vi "Define Mask.vi"(8 "error in (no error)":errorcluster, 11 "FPGA Image":T3(plugin-control)=refnum) -> (0 "error out":errorcluster)   [LabVIEW 2013]
doc: "GUI for selecting a part type and starting a batch process\nPart types list is passed in from caller.\nReturns when Start or Cancel is pressed."
uses:
  Sectors/Number of Wing Sector.ctl
  Mask ROI FG Enum.ctl
  Mask ROI Cluster.ctl
  Common/File IO/INI/Read write mode.ctl
  Message Passing/MsgQ Loops enum.ctl
  System Status/Status FG Enum.ctl
  Common/State Machines/State Machine Lib.lvlib
  Common/GUI/GUI.lvlib
  <vilib>/vision/NI_Vision_Development_Module.lvlib
  Image Processing.lvlib
  Message Passing/Main MsgQ.lvlib
panel:
  in  "Calculate BG":bool
  in  "Load Current Mask":bool
  out "Right ROI":T1 {"Contours"."Type" items=["No Selection", "Point", "Line", "Rectangle", "Oval", "Polygon", "Freehand Region", "Annulus", "Unused2", "Unused3", "Broken Line", "Freehand Line", "Rotated Rectangle"]}
  out "Left ROI":T1 {"Contours"."Type" items=["No Selection", "Point", "Line", "Rectangle", "Oval", "Polygon", "Freehand Region", "Annulus", "Unused2", "Unused3", "Broken Line", "Freehand Line", "Rotated Rectangle"]}
  out "[Avg BG]":dbl[](array[numeric])
  in  "NumWingSectors":T2=1 items=["1"=1, "2"=2, "4"=4, "8"=8, "16"=16]
  out "State":string
  in  "Exit":bool
  in  "Save Mask":bool
  out "combo mask":T3(plugin-control)
  out "right mask":T3(plugin-control)
  out "right masked image":T3(plugin-control)
  out "right annulus":T4={"Center X"=929, "Center Y"=663, "Inner Radius"=200, "Outer Radius"=405, "Start Angle"=90.0, "End Angle"=180.0} {"End Angle" format="%.2f"; "Start Angle" format="%.2f"; "Center X" scale=0.0..1024.0}
  out "left mask":T3(plugin-control)
  out "left masked image":T3(plugin-control)
  out "left annulus":T4={"Center X"=929, "Center Y"=663, "Inner Radius"=200, "Outer Radius"=405, "Start Angle"=90.0, "End Angle"=180.0} {"End Angle" format="%.2f"; "Start Angle" format="%.2f"; "Center X" scale=0.0..1024.0}
  in  "Accept Threshold":bool
  out "Processed Image":T3(plugin-control)
  in  "Threshold Range":cluster{"Lower value":dbl, "Upper value":dbl}={"Lower value"=106.82432432432432, "Upper value"=255.0} {"Upper value" min=0.0 max=255.0 scale=0.0..255.0; "Lower value" min=0.0 max=255.0 scale=0.0..255.0}
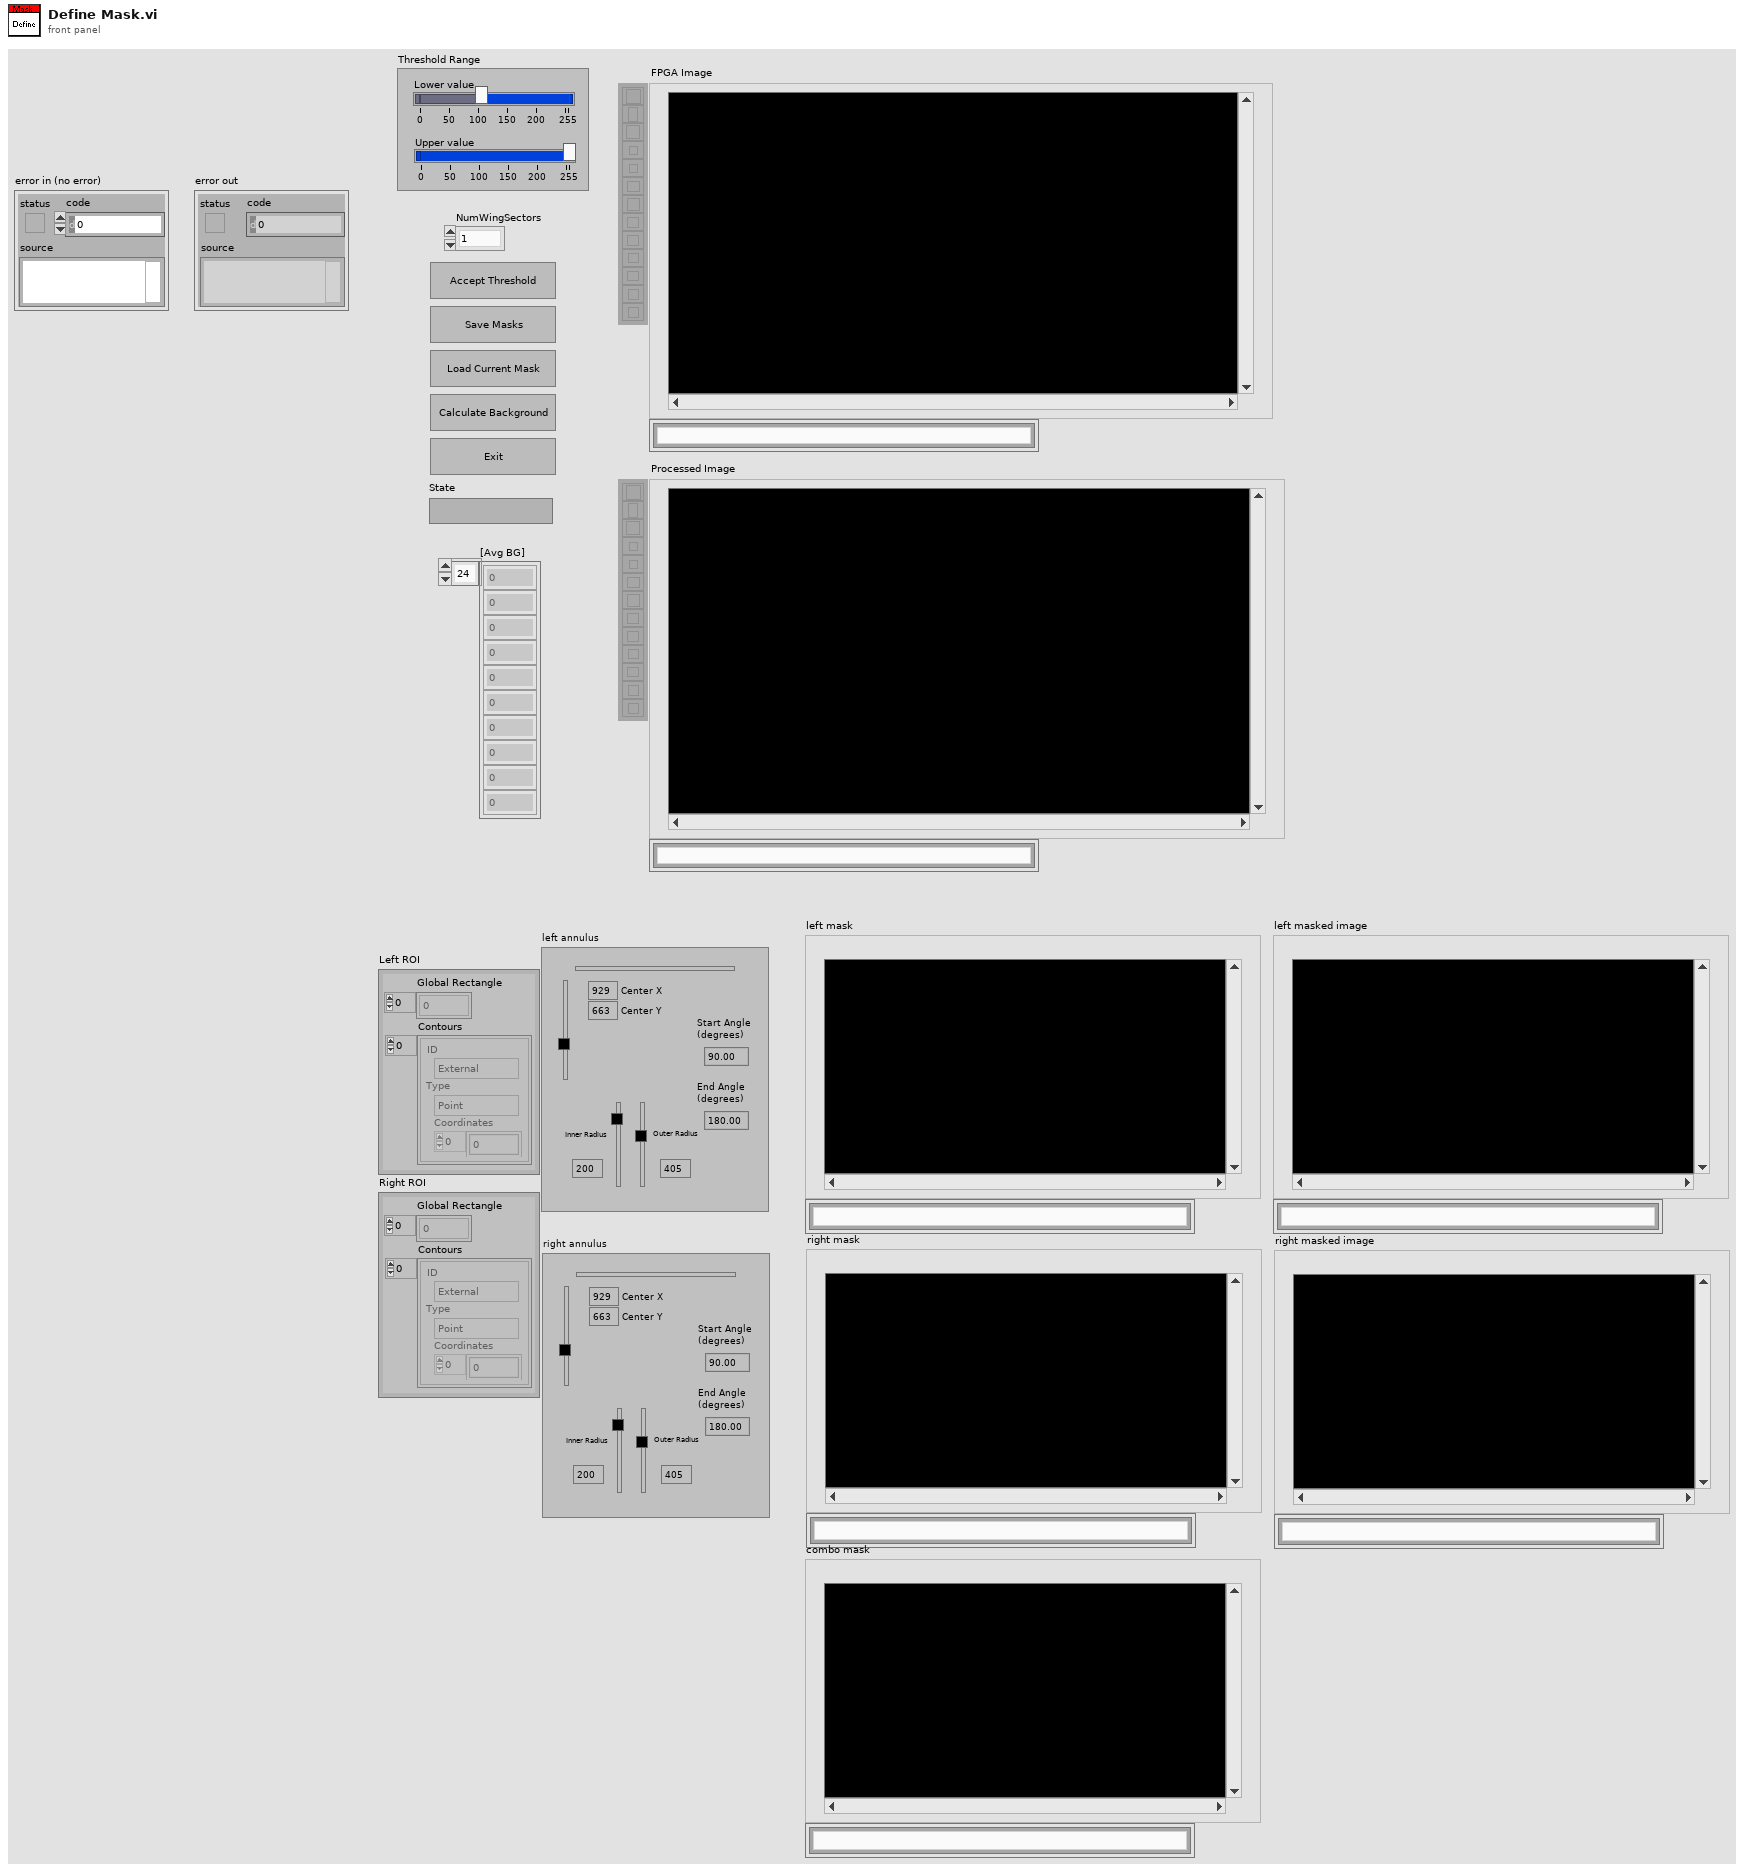
[diagram p1: front panel]
types:
  T1 = typedef "ROI Descriptor" = cluster{"Global Rectangle":i32[], "Contours":cluster{"ID":enum32{"External", "Internal"}, "Type":u32, "Coordinates":i32[]}[]}
  T2 = typedef "Number of Wing Sector.ctl" = u8
  T3 = typedef "IMAQ Image.ctl" = refnum<image>
  T4 = typedef "IMAQ Circle" = cluster{"Center X":i32, "Center Y":i32, "Inner Radius":i32, "Outer Radius":i32, "Start Angle":dbl, "End Angle":dbl}
  T5 = typedef "State Machine Lib.lvlib/STATE cluster.ctl" = cluster{"State":string, "Parameters":variant}
  T6 = typedef "Mask ROI FG Enum.ctl" = enum16{"Read", "Write"}
  T7 = typedef "Main MsgQ.lvlib/MsgQ Loops enum.ctl" = enum16{"User Interface", "Image Acq"}
  T8 = typedef "Read write mode.ctl" = enum16{"Read", "Write"}
  T9 = typedef "Mask ROI Cluster.ctl" = cluster{"left annulus":T4, "right annulus":T4, "Threshold Range":cluster{"Lower value":dbl, "Upper value":dbl}, "[Avg BG]":u8[], "Number of Sectors":u8, "Left ROI":T1, "Right ROI":T1, "Left Start Angle Duty Cycle":fxp<+,8,0>, "Left End Angle Duty Cycle":fxp<+,8,0>, "Right End Angle Duty Cycle":fxp<+,8,0>, "Right Start Angle Duty Cycle":fxp<+,8,0>, "[Sector ROIs]":T1[]}
  T10 = typedef "Status FG Enum.ctl" = enum16{"Reset", "Read", "Write"}
  T11 = typedef "Sector Parameter Cluster.ctl" = cluster{"Start Angle":fxp<+/-,17,2>, "End Angle":fxp<+/-,17,2>, "Inner Radius":u16, "Outter Radius":u16, "Hinge X":u16, "Hinge Y":u16, "NumWingSectors":u8}
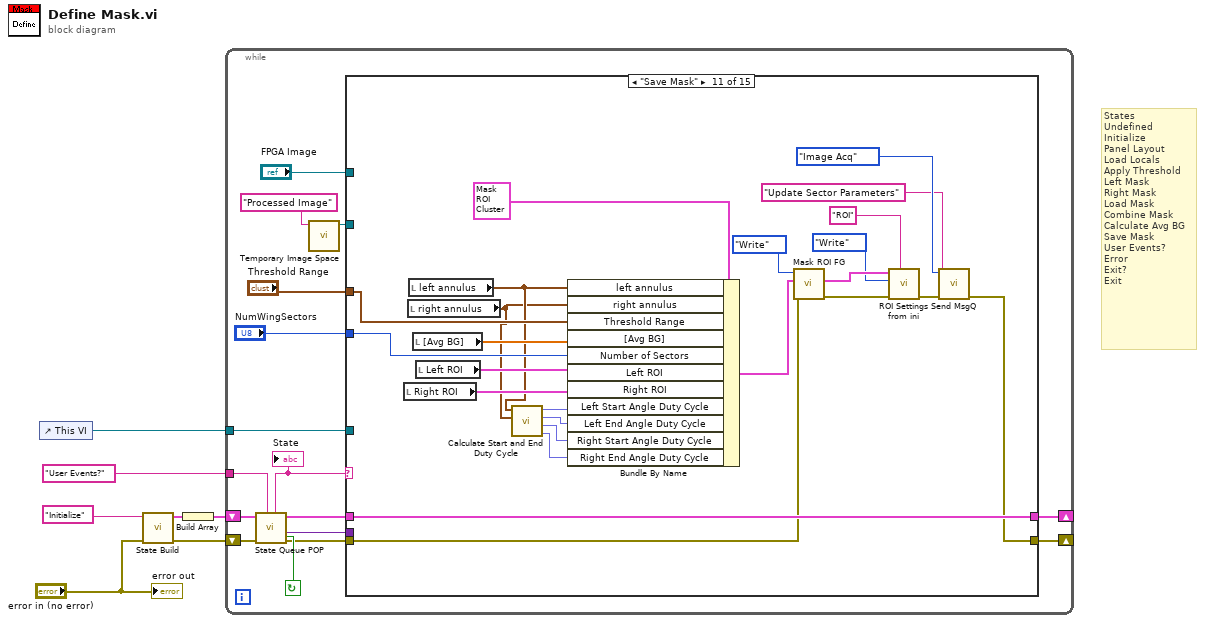
[diagram p0: block diagram]
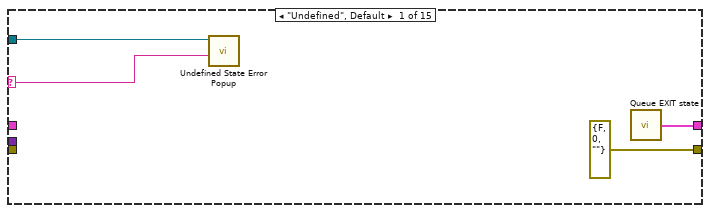
[diagram p2: hidden frame]
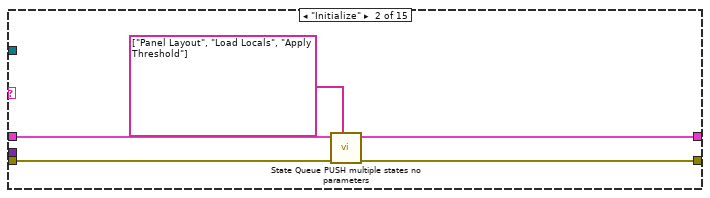
[diagram p3: hidden frame]
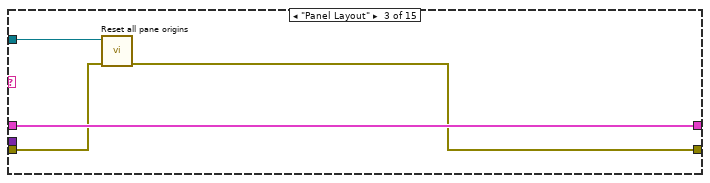
[diagram p4: hidden frame]
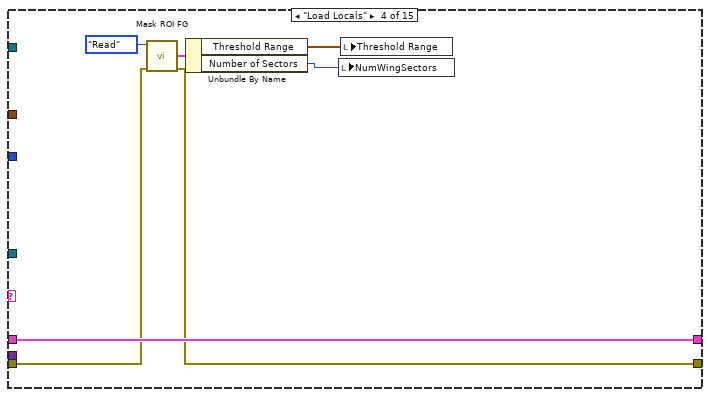
[diagram p5: hidden frame]
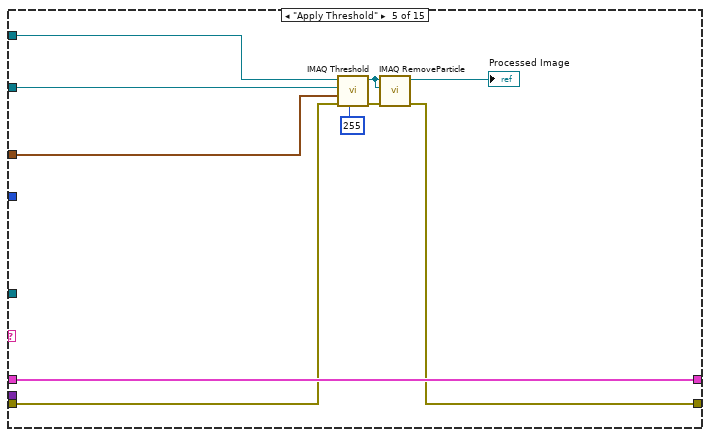
[diagram p6: hidden frame]
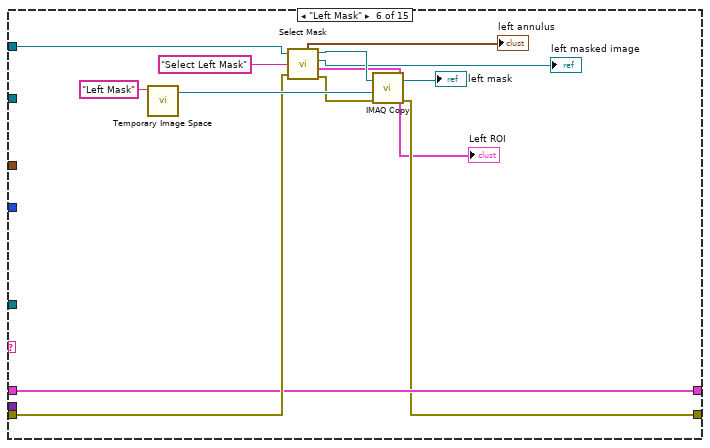
[diagram p7: hidden frame]
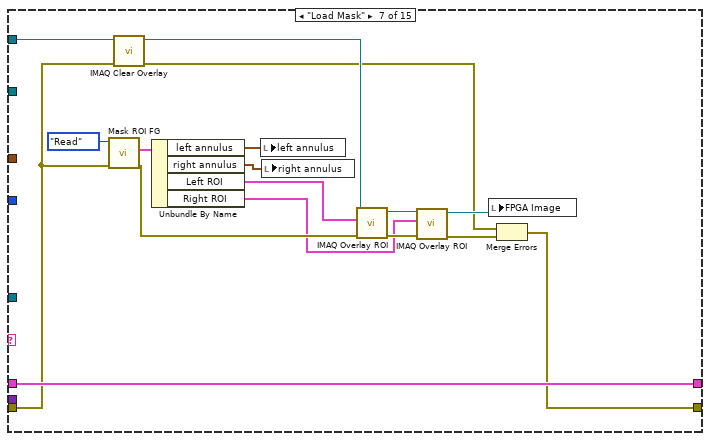
[diagram p8: hidden frame]
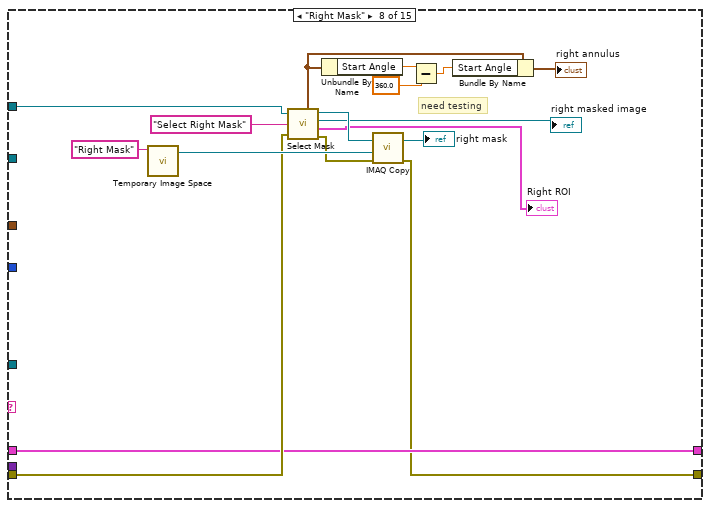
[diagram p9: hidden frame]
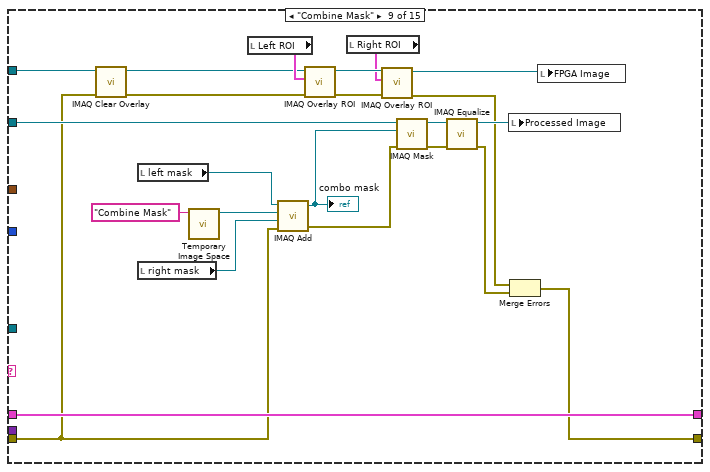
[diagram p10: hidden frame]
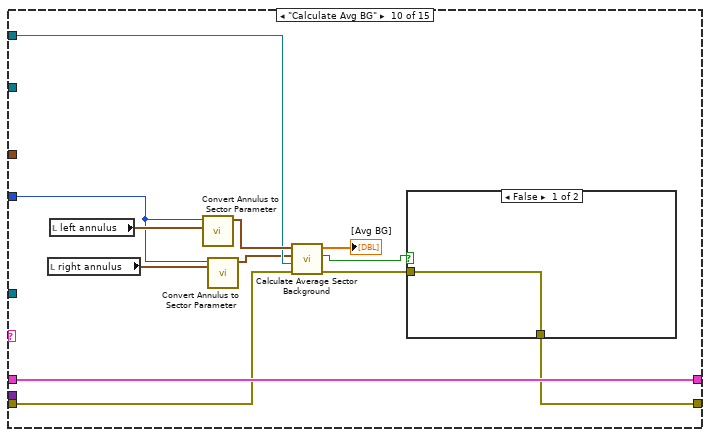
[diagram p11: hidden frame]
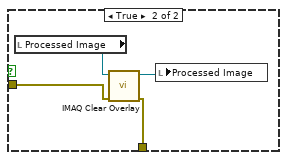
[diagram p12: hidden frame]
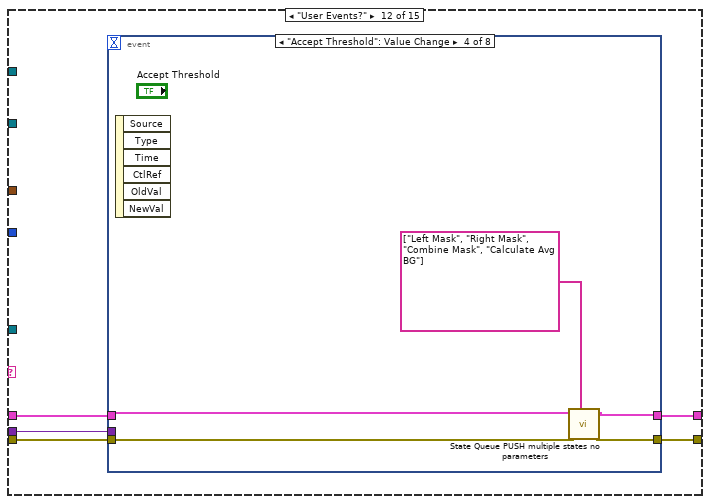
[diagram p13: hidden frame]
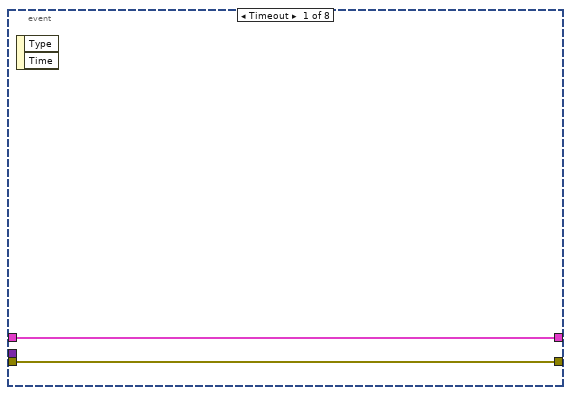
[diagram p14: hidden frame]
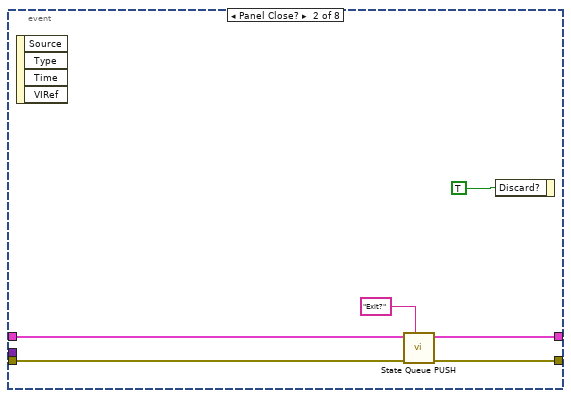
[diagram p15: hidden frame]
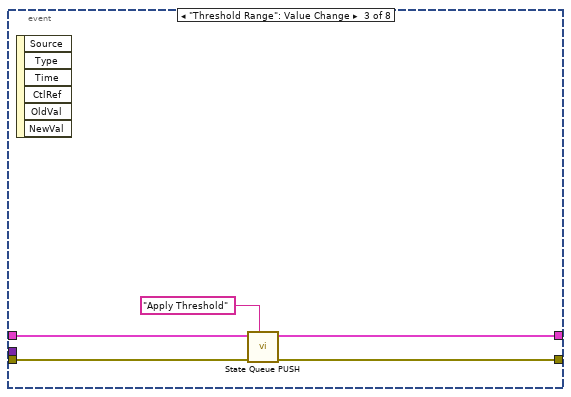
[diagram p16: hidden frame]
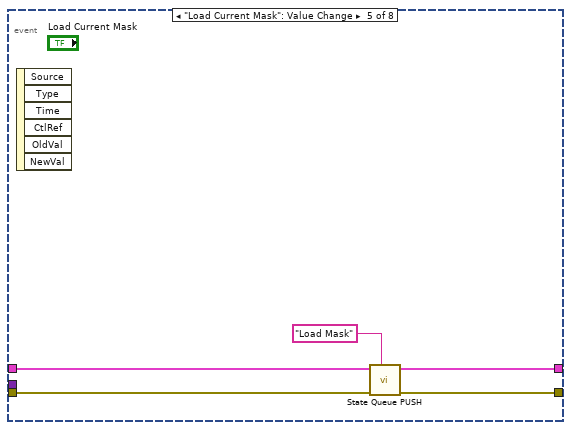
[diagram p17: hidden frame]
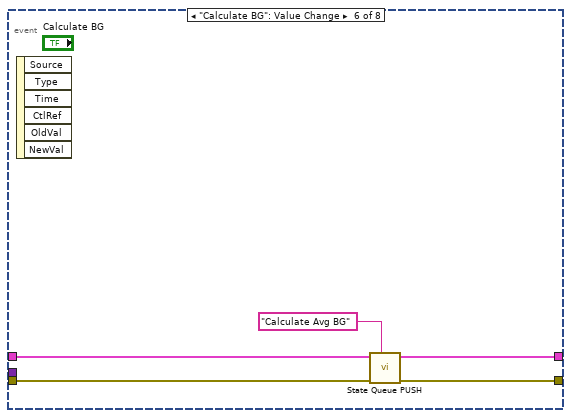
[diagram p18: hidden frame]
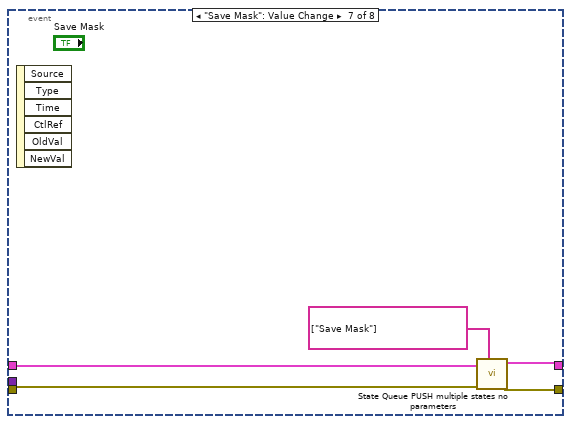
[diagram p19: hidden frame]
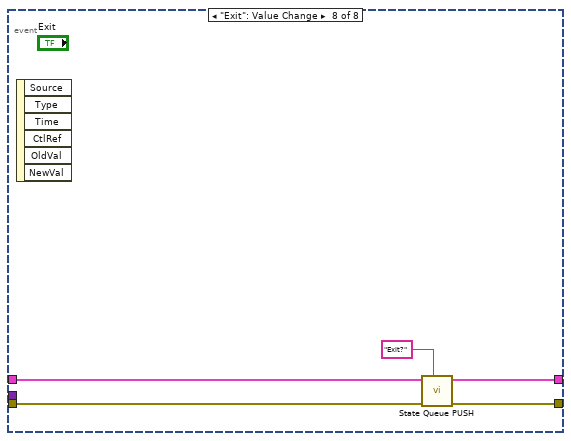
[diagram p20: hidden frame]
diagram:
  # "States\nUndefined\nInitialize\nPanel Layout\nLoad Locals\nApply Threshold\nLeft Mask\nRight Mask\nLoad Mask\nCombine Mask\nCalculate Avg BG\nSave Mask\nUser Events?\nError\nExit?\nExit"
  n1 = control-ref of="This VI"() -> (w6:refnum<vi>)
  n2 = call "State Build.vi"("error in (no error)"="error in (no error)", "State"="Initialize") -> ("error out"=w3:errorcluster, "State Out"=w4:T5)  [unwired: 8 in]
  n3 = Build Array(w4) -> (w5:T5[])
  n4 = while {
    shift-right: [w14] -> _
    shift-left: w3 -> [w22]
    shift-right: [w13] -> _
    shift-left: w5 -> [w20]
    tunnel: "User Events?" ("Default state") -> [w21]
    tunnel: w6 -> [w16]
    stop <- w23 continue-if-true
    n5 = call "State Queue POP.vi"("Default state"=w21, "error in (no error)"=w22, "State que in"=w20) -> ("error out"=w19:errorcluster, "Parameters"=w15:variant, "State que out"=w18:T5[], "Not Exit?"=w23:bool, "State case out"=w17:string)  [unwired: 4 out]
    "State" <- w17
    n6 = call "Temporary Image Space.vi"("Image Name"="Processed Image") -> ("Image Out"=w10:T3)  [unwired: 10 in]
    n7 = case shown="\"Save Mask\"" w17 {
      selector: w17 -> [w24 _ _ _ _ _ _ _ _ _ _ _ _ _ _]
      tunnel: w19 -> [_ w30 w34 w38 w48 w59 w70 w93 w106 w134 w159 w168 w208 w222 _]
      tunnel: w18 -> [_ w32 w36 w43 w49 w58 w82 w92 w113 w135 w164 w169 _ w216 w224]
      tunnel: w16 -> [w25 _ w35 _ _ _ _ _ _ _ _ _ _ _ _]
      tunnel: w15 -> [_ _ _ _ _ _ _ _ _ _ _ w167 _ _ _]
      tunnel: [errorcluster {"status"=FALSE, "code"=0, "source"=""} ("error out") w31 w33 w37 w47 w57 w67 w91 w103 w125 w149 w166 errorcluster {"status"=FALSE, "code"=0, "source"=""} ("error out") w222 errorcluster {"status"=FALSE, "code"=0, "source"=""} ("error out")] -> w14
      tunnel: [w27 w28 w36 w43 w49 w58 w82 w92 w113 w135 w164 w165 w213 w215 w224] -> w13
      tunnel: "Threshold Range" -> [_ _ _ _ w46 _ _ _ _ _ w161 _ _ _ _]
      tunnel: "FPGA Image" -> [_ _ _ _ w45 w60 w72 w94 w108 w131 _ _ _ _ _]
      tunnel: w10 -> [_ _ _ _ w44 _ _ _ w116 _ _ _ _ _ _]
      tunnel: "NumWingSectors" -> [_ _ _ _ _ _ _ _ _ w129 w157 _ _ _ _]
      frame "Undefined", Default {
        n8 = call "Undefined State Error Popup.vi"("String"=w24, "This VI (Caller if unwired)"=w25) -> ()  [unwired: 10 out]
        n9 = call "Queue EXIT state.vi"() -> ("Exit State Q"=w27:T5[])  [unwired: 1 in]
      }
      frame "Initialize" {
        n10 = call "State Queue PUSH multiple states no parameters.vi"("States to queue"=string[] ["Panel Layout", "Load Locals", "Apply Threshold"], "error in (no error)"=w30, "State que in"=w32) -> ("error out"=w31:errorcluster, "State que out"=w28:T5[])  [unwired: 1 in, 6 out]
      }
      frame "Panel Layout" {
        n11 = call "Reset all pane origins.vi"("error in (no error"=w34, "Vi Ref In"=w35) -> ("error out"=w33:errorcluster)  [unwired: 9 out]
      }
      frame "Load Locals" {
        n12 = call "Mask ROI FG.vi"("error in (no error)"=w38, "Operation"=Mask_ROI_FG_Enum."Read") -> ("error out"=w37:errorcluster, "Mask ROI Out"=w41:T9)  [unwired: 8 in]
        n13 = Unbundle By Name(w41) -> ("Threshold Range"=w40:cluster{"Lower value":dbl, "Upper value":dbl}, "Number of Sectors"=w39:u8)
        n14 = local write "NumWingSectors"(w39) -> ()
        n15 = local write "Threshold Range"(w40) -> ()
      }
      frame "Apply Threshold" {
        n16 = call "IMAQ Threshold"("Replace Value"=u8 255, "error in (no error)"=w48, "Range"=w46, "Image Dst"=w44, "Image Src"=w45) -> ("error out"=w51:errorcluster, "Image Dst Out"=w53:T3)  [unwired: 1 in, 4 out]
        n17 = call "IMAQ RemoveParticle"("error in (no error)"=w51, "Image Dst"=w53, "Image Src"=w53) -> ("error out"=w47:errorcluster, "Image Dst Out"=→"Processed Image":T3)  [unwired: 4 in, 3 out]
      }
      frame "Left Mask" {
        n18 = call "Temporary Image Space.vi"("Image Name"="Left Mask") -> ("Image Out"=w61:T3)  [unwired: 10 in]
        n19 = call "Select Mask.vi"("error in"=w59, "Prompt"="Select Left Mask", "Read \nImage"=w60) -> ("error out"=w56:errorcluster, "ROI Descriptor Out"=→"Left ROI":T1, "Masked \nImage"=→"left masked image":T3, "Annulus"=→"left annulus":T4, "mask"=w64:T3)  [unwired: 1 out]
        n20 = call "IMAQ Copy"("error in (no error)"=w56, "Image Dst"=w61, "Image Src"=w64) -> ("error out"=w57:errorcluster, "Image Dst Out"=→"left mask":T3)  [unwired: 3 in]
      }
      frame "Load Mask" {
        n21 = call "Mask ROI FG.vi"("error in (no error)"=w70, "Operation"=Mask_ROI_FG_Enum."Read") -> ("error out"=w75:errorcluster, "Mask ROI Out"=w81:T9)  [unwired: 8 in]
        n22 = call "IMAQ Clear Overlay"("error in (no error)"=w70, "Image"=w72) -> ("error out"=w69:errorcluster, "Image Out"=w71:T3)  [unwired: 8 in]
        n23 = Unbundle By Name(w81) -> ("left annulus"=w80:T4, "right annulus"=w79:T4, "Left ROI"=w74:T1, "Right ROI"=w73:T1)
        n24 = local write "left annulus"(w80) -> ()
        n25 = local write "right annulus"(w79) -> ()
        n26 = call "IMAQ Overlay ROI"("error in (no error)"=w75, "ROI Descriptor"=w74, "Image"=w71) -> ("error out"=w76:errorcluster, "Image Out"=w78:T3)  [unwired: 7 in]
        n27 = call "IMAQ Overlay ROI"("error in (no error)"=w76, "ROI Descriptor"=w73, "Image"=w78) -> ("error out"=w68:errorcluster, "Image Out"=w77:T3)  [unwired: 7 in]
        n28 = local write "FPGA Image"(w77) -> ()
        n29 = Merge Errors(w69, w68) -> (w67:errorcluster)
      }
      frame "Right Mask" {
        # "need testing"
        n30 = call "Temporary Image Space.vi"("Image Name"="Right Mask") -> ("Image Out"=w95:T3)  [unwired: 10 in]
        n31 = call "Select Mask.vi"("error in"=w93, "Prompt"="Select Right Mask", "Read \nImage"=w94) -> ("error out"=w90:errorcluster, "ROI Descriptor Out"=→"Right ROI":T1, "Masked \nImage"=→"right masked image":T3, "Annulus"=w84:T4, "mask"=w98:T3)  [unwired: 1 out]
        n32 = Unbundle By Name(w84) -> ("Start Angle"=w89:dbl)
        n33 = call "IMAQ Copy"("error in (no error)"=w90, "Image Dst"=w95, "Image Src"=w98) -> ("error out"=w91:errorcluster, "Image Dst Out"=→"right mask":T3)  [unwired: 3 in]
        n34 = Subtract(x=w89, y=360.0) -> (x-y=w87:dbl)
        n35 = Bundle By Name(cluster=w84, "Start Angle"=w87) -> (→"right annulus":T4)
      }
      frame "Combine Mask" {
        n36 = call "IMAQ Clear Overlay"("error in (no error)"=w106, "Image"=w108) -> ("error out"=w105:errorcluster, "Image Out"=w107:T3)  [unwired: 8 in]
        n37 = local read "left mask"() -> (w118:T3)
        n38 = local read "right mask"() -> (w117:T3)
        n39 = call "Temporary Image Space.vi"("Image Name"="Combine Mask") -> ("Image Out"=w120:T3)  [unwired: 10 in]
        n40 = local read "Left ROI"() -> (w112:T1)
        n41 = call "IMAQ Add"("Image Src A"=w118, "Image Dst"=w120, "Image Src B"=w117, "error in (no error)"=w106) -> ("Image Dst Out"=w121:T3, "error out"=w114:errorcluster)  [unwired: 3 in]
        "combo mask" <- w121
        n42 = call "IMAQ Overlay ROI"("error in (no error)"=w105, "ROI Descriptor"=w112, "Image"=w107) -> ("error out"=w104:errorcluster, "Image Out"=w111:T3)  [unwired: 7 in]
        n43 = local read "Right ROI"() -> (w110:T1)
        n44 = call "IMAQ Overlay ROI"("error in (no error)"=w104, "ROI Descriptor"=w110, "Image"=w111) -> ("error out"=w101:errorcluster, "Image Out"=w109:T3)  [unwired: 7 in]
        n45 = call "IMAQ Mask"("error in (no error)"=w114, "Image Mask"=w121, "Image Src"=w116) -> ("error out"=w122:errorcluster, "Image Dst Out"=w123:T3)  [unwired: 1 in, 1 out]
        n46 = call "IMAQ Equalize"("error in (no error)"=w122, "Image Src"=w123) -> ("error out"=w102:errorcluster, "Image Dst Out"=w115:T3)  [unwired: 4 in, 4 out]
        n47 = local write "Processed Image"(w115) -> ()
        n48 = Merge Errors(w101, w102) -> (w103:errorcluster)
        n49 = local write "FPGA Image"(w109) -> ()
      }
      frame "Calculate Avg BG" {
        n50 = local read "right annulus"() -> (w128:T4)
        n51 = local read "left annulus"() -> (w133:T4)
        n52 = call "Convert Annulus to Sector Parameter.vi"("Annulus"=w133, "NumWingSectors"=w129) -> ("Sector Parameter"=w132:T11)  [unwired: 9 in]
        n53 = call "Convert Annulus to Sector Parameter.vi"("Annulus"=w128, "NumWingSectors"=w129) -> ("Sector Parameter"=w127:T11)  [unwired: 9 in]
        n54 = call "Calculate Average Sector Background.vi"("error in (no error)"=w134, "Image"=w131, "Right Sector Parameters"=w127, "Left Sector Parameters"=w132) -> ("error out"=w126:errorcluster, "Canceled?"=w124:bool, "[Avg BG]"=→"[Avg BG]":dbl[])  [unwired: 5 in]
        n55 = case shown="False" w124 {
          tunnel: w126 -> [w136 w139]
          tunnel: [w136 w138] -> w125
          frame False {
          }
          frame True {
            n56 = local read "Processed Image"() -> (w140:T3)
            n57 = call "IMAQ Clear Overlay"("error in (no error)"=w139, "Image"=w140) -> ("error out"=w138:errorcluster, "Image Out"=w137:T3)  [unwired: 8 in]
            n58 = local write "Processed Image"(w137) -> ()
          }
        }
      }
      frame "Save Mask" {
        n59 = local read "Right ROI"() -> (w147:T1)
        n60 = local read "right annulus"() -> (w145:T4)
        n61 = local read "left annulus"() -> (w146:T4)
        n62 = local read "[Avg BG]"() -> (w158:dbl[])
        n63 = local read "Left ROI"() -> (w148:T1)
        n64 = call "Calculate Start and End Duty Cycle.vi"("right annulus"=w145, "left annulus"=w146) -> ("Right End Angle Duty Cycle"=w141:fxp<+,8,0>, "Right Start Angle Duty Cycle"=w142:fxp<+,8,0>, "Left End Angle Duty Cycle"=w143:fxp<+,8,0>, "Left Start Angle Duty Cycle"=w144:fxp<+,8,0>)  [unwired: 6 in]
        n65 = Bundle By Name(cluster=T9 {"left annulus"={"Center X"=929, "Center Y"=663, "Inner Radius"=200, "Outer Radius"=405, "Start Angle"=90.0, "End Angle"=180.0}, "right annulus"={"Center X"=929, "Center Y"=663, "Inner Radius"=200, "Outer Radius"=405, "Start Angle"=90.0, "End Angle"=180.0}, "Threshold Range"={"Lower value"=106.82432432432432, "Upper value"=255.0}, "[Avg BG]"=[], "Number of Sectors"=0, "Left ROI"={"Global Rectangle"=[], "Contours"=[]}, "Right ROI"={"Global Rectangle"=[], "Contours"=[]}, "Left Start Angle Duty Cycle"=0.0, "Left End Angle Duty Cycle"=0.0, "Right End Angle Duty Cycle"=0.0, "Right Start Angle Duty Cycle"=0.0, "[Sector ROIs]"=[]} ("Mask ROI In"), "left annulus"=w146, "right annulus"=w145, "Threshold Range"=w161, "[Avg BG]"=w158, "Number of Sectors"=w157, "Left ROI"=w148, "Right ROI"=w147, "Left Start Angle Duty Cycle"=w144, "Left End Angle Duty Cycle"=w143, "Right Start Angle Duty Cycle"=w142, "Right End Angle Duty Cycle"=w141) -> (w160:T9)
        n66 = call "Mask ROI FG.vi"("error in (no error)"=w159, "Mask ROI In"=w160, "Operation"=Mask_ROI_FG_Enum."Write") -> ("error out"=w154:errorcluster, "Mask ROI Out"=w156:T9)  [unwired: 7 in]
        n67 = call "ROI Settings from ini.vi"("Section"="ROI", "error in (no error)"=w154, "Operation"=Read_write_mode."Write", "Mask ROI In"=w156) -> ("error out"=w150:errorcluster)  [unwired: 5 in, 2 out]
        n68 = call "Send MsgQ.vi"("error in (no error)"=w150, "Message String"="Update Sector Parameters", "Send to MsgQ"=MsgQ_Loops_enum."Image Acq") -> ("error out"=w149:errorcluster)  [unwired: 8 in]
      }
      frame "User Events?" {
        n69 = event shown="[3] \"Accept Threshold\": Value Change" {
          selector: _ -> [_ _ _ _ _ _ _ _]
          dyn-events: _ -> [_ _ _ _ _ _ _ _]
          timeout: _ -> [_ _ _ _ _ _ _ _]
          tunnel: w169 -> [w170 w176 w182 w185 w191 w196 w201 w204]
          tunnel: w168 -> [w171 w175 w181 w183 w188 w193 w198 w205]
          tunnel: w167 -> [_ _ _ _ _ _ _ _]
          tunnel: [w171 w173 w179 w186 w189 w194 w199 w206] -> w166
          tunnel: [w170 w174 w180 w187 w190 w195 w200 w207] -> w165
          event Timeout {
            n70 = event-data() -> ()  [unwired: 3 out]
          }
          event Panel Close? {
            n71 = event-data() -> ()  [unwired: 5 out]
            n72 = call "State Queue PUSH.vi"("State case"="Exit?", "error in (no error)"=w175, "State que in"=w176) -> ("error out"=w173:errorcluster, "State que out"=w174:T5[])  [unwired: 2 in, 5 out]
            n73 = event-data("Discard?"=TRUE) -> ()  [unwired: 1 in, 1 out]
          }
          event "Threshold Range": Value Change {
            n74 = event-data() -> ()  [unwired: 7 out]
            n75 = call "State Queue PUSH.vi"("State case"="Apply Threshold", "error in (no error)"=w181, "State que in"=w182) -> ("error out"=w179:errorcluster, "State que out"=w180:T5[])  [unwired: 2 in, 5 out]
          }
          event "Accept Threshold": Value Change {
            n76 = event-data() -> ()  [unwired: 7 out]
            n77 = call "State Queue PUSH multiple states no parameters.vi"("States to queue"=string[] ["Left Mask", "Right Mask", "Combine Mask", "Calculate Avg BG"], "error in (no error)"=w183, "State que in"=w185) -> ("error out"=w186:errorcluster, "State que out"=w187:T5[])  [unwired: 7 in]
          }
          event "Load Current Mask": Value Change {
            n78 = event-data() -> ()  [unwired: 7 out]
            n79 = call "State Queue PUSH.vi"("State case"="Load Mask", "error in (no error)"=w188, "State que in"=w191) -> ("error out"=w189:errorcluster, "State que out"=w190:T5[])  [unwired: 2 in, 5 out]
          }
          event "Calculate BG": Value Change {
            n80 = event-data() -> ()  [unwired: 7 out]
            n81 = call "State Queue PUSH.vi"("State case"="Calculate Avg BG", "error in (no error)"=w193, "State que in"=w196) -> ("error out"=w194:errorcluster, "State que out"=w195:T5[])  [unwired: 2 in, 5 out]
          }
          event "Save Mask": Value Change {
            n82 = event-data() -> ()  [unwired: 7 out]
            n83 = call "State Queue PUSH multiple states no parameters.vi"("States to queue"=string[] ["Save Mask"], "error in (no error)"=w198, "State que in"=w201) -> ("error out"=w199:errorcluster, "State que out"=w200:T5[])  [unwired: 7 in]
          }
          event "Exit": Value Change {
            n84 = event-data() -> ()  [unwired: 7 out]
            n85 = call "State Queue PUSH.vi"("State case"="Exit?", "error in (no error)"=w205, "State que in"=w204) -> ("error out"=w206:errorcluster, "State que out"=w207:T5[])  [unwired: 7 in]
          }
        }
      }
      frame "Error" {
        # "DEFAULT IS \nTO CLEAR ERROR\nAND EXIT"
        n86 = Unbundle By Name(w208) -> ("source"=w211:string)
        n87 = Concatenate Strings("Error: " ("string"), w211) -> (w210:string)
        n88 = call "Status FG.vi"("Status In"=w210, "Operation"=Status_FG_Enum."Write") -> ()  [unwired: 8 in, 2 out]
        n89 = call <vilib>:"Clear Errors.vi"("error in (no error)"=w208) -> ()  [unwired: 7 out]
        n90 = call "Queue EXIT state.vi"() -> ("Exit State Q"=w213:T5[])  [unwired: 1 in]
      }
      frame "Exit?" {
        n91 = Two Button Dialog(message="Exit?", 1:"No" ("F button name (\"Cancel\")"), 2:"Yes" ("T button name (\"OK\")")) -> (T button?=w218:bool)
        n92 = call "Queue EXIT state.vi"() -> ("Exit State Q"=w217:T5[])  [unwired: 1 in]
        n93 = Select(t=w217, s=w218, f=w216) -> (s? t:f=w215:T5[])
      }
      frame "Exit" {
      }
    }
  }
  "error out" <- "error in (no error)"
